vi "test File With Trailing Period Gets Extension.vi"(8 "error in (no error)":errorcluster, 11 "TestCase in":refnum<class "Build Linux Log File Path.lvclass">) -> (0 "error out":errorcluster, 3 "TestCase out":refnum<class "Build Linux Log File Path.lvclass">)   [LabVIEW 2024, in "Build Linux Log File Path.lvclass"]
uses:
  Build Linux Log File Path.lvclass
  <vilib>/addons/_JKI Toolkits/VI Tester/TestCase.llb/TestCase.lvclass
  C:/Program Files/National Instruments/LabVIEW 2024/vi.lib/addons/_JKI Toolkits/VI Tester/TestCase.llb/TestCase.lvclass
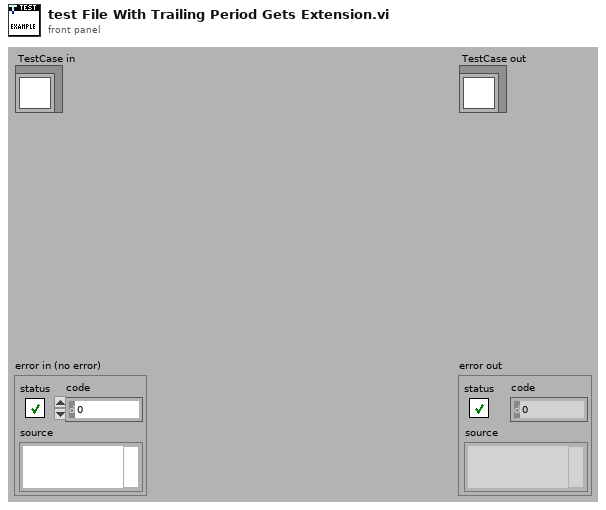
[diagram p1: front panel]
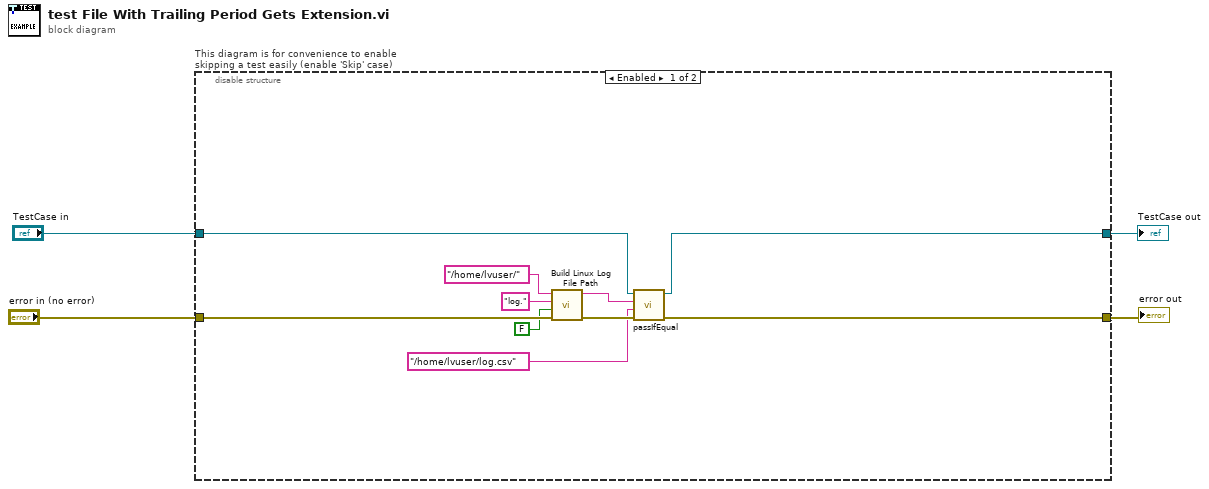
[diagram p0: block diagram]
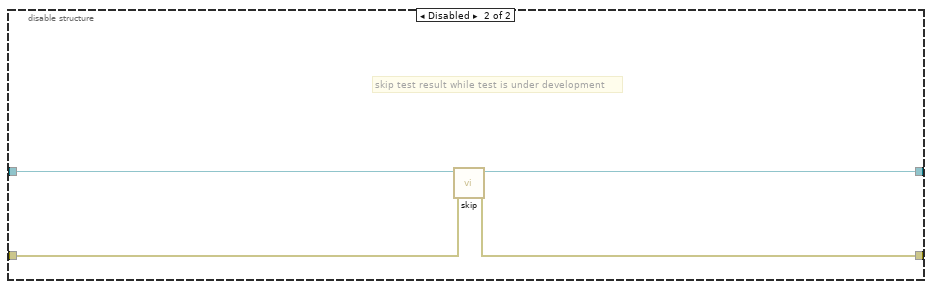
[diagram p2: hidden frame]
diagram:
  n1 = disable-structure "This diagram is for convenience to enable skipping a test easily (enable 'Skip' case)" shown="Enabled" {
    disable-tunnel: "TestCase in" -> [w13 w18]
    disable-tunnel: [w8 w16] -> w1
    disable-tunnel: [w7 w17] -> w3
    disable-tunnel: "error in (no error)" -> [w14 w15]
    frame Enabled {
      n2 = call "Build Linux Log File Path.vi"("error in (no error)"=w14, "Timestamp"=FALSE, "Name"="log.", "Log File Directory"="/home/lvuser/") -> ("error out"=w12:errorcluster, "Log File Path"=w6:string)  [unwired: 6 in]
      n3 = call-dynamic "passIfEqual.vi"("error in (no error)"=w12, "y"="/home/lvuser/log.csv", "x"=w6, "TestCase in"=w13) -> ("error out"=w7:errorcluster, "TestCase out"=w8:refnum<class "Build Linux Log File Path.lvclass">)  [unwired: 6 in]
    }
    frame Disabled {
      # "skip test result while test is under development"
      n4 = call <vilib>:"skip.vi"("error in (no error)"=w15, "TestCase in"=w18) -> ("error out"=w17:errorcluster, "TestCase out"=w16:refnum<class "Build Linux Log File Path.lvclass">)  [unwired: 8 in]
    }
  }
  "error out" <- w3
  "TestCase out" <- w1
